vi "bangBangMove.vi"(10 "numRoundingPts":u16, 11 "numPts":u16) -> (3 "roundedHalfTriangle":dbl[](array[numeric]))   [LabVIEW 2016]
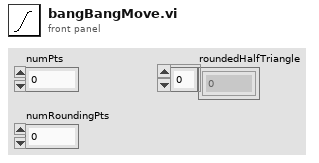
[diagram p1: front panel]
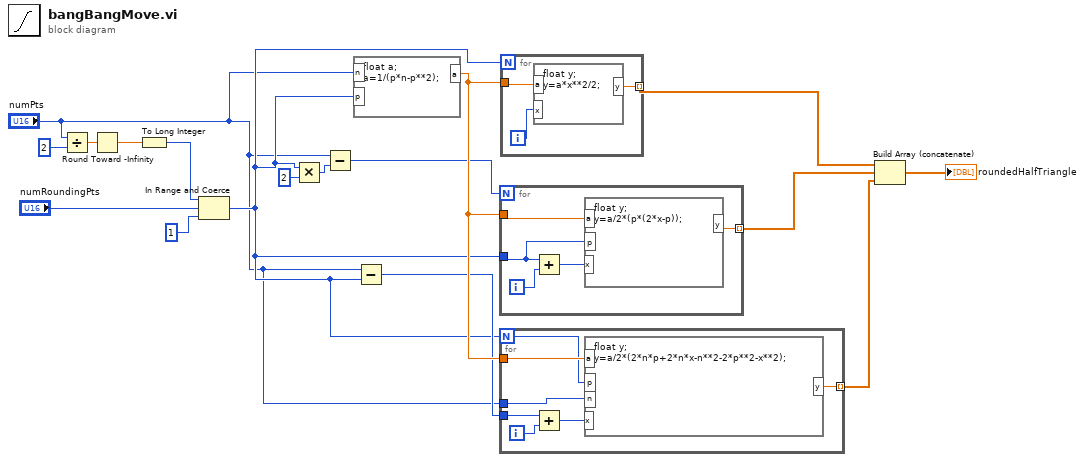
[diagram p0: block diagram]
diagram:
  n1 = Divide(x="numPts", y=u16 2) -> (x/y=w4:dbl)
  n2 = Round Toward -Infinity(1:w4) -> (0:w3:dbl)
  n3 = To Long Integer(number=w3) -> (32bit integer=w1:i32)
  n4 = In Range and Coerce(upper limit=w1, x="numRoundingPts", lower limit=1) -> (coerced(x)=w7:i32)  [unwired: 1 out]
  n5 = Multiply(x=w7, y=u16 2) -> (x*y=w9:i32)
  n6 = Subtract(x="numPts", y=w9) -> (x-y=w10:i32)
  n7 = formula code="float a;\na=1/(p*n-p**2);"("n"="numPts", "p"=w7) -> ("a"=w14:dbl)
  n8 = Subtract(x="numPts", y=w7) -> (x-y=w13:i32)
  n9 = for {
    N: w10 -> [_]
    tunnel: w14 -> [w22]
    tunnel: [w20] -> w12 mode=indexing
    tunnel: w7 -> [w18]
    i -> [w21]
    n10 = Add(x=w18, y=w21) -> (x+y=w19:i32)
    n11 = formula code="float y;\ny=a/2*(p*(2*x-p));"("a"=w22, "x"=w19, "p"=w18) -> ("y"=w20:dbl)
  }
  n12 = for {
    N: w7 -> [w23]
    tunnel: w14 -> [w29]
    tunnel: [w27] -> w15 mode=indexing
    tunnel: w13 -> [w25]
    tunnel: "numPts" -> [w24]
    i -> [w28]
    n13 = Add(x=w25, y=w28) -> (x+y=w26:i32)
    n14 = formula code="float y;\ny=a/2*(2*n*p+2*n*x-n**2-2*p**2-x**2);"("a"=w29, "x"=w26, "n"=w24, "p"=w23) -> ("y"=w27:dbl)
  }
  n15 = for {
    N: w7 -> [_]
    tunnel: w14 -> [w32]
    tunnel: [w30] -> w11 mode=indexing
    i -> [w31]
    n16 = formula code="float y;\ny=a*x**2/2;"("a"=w32, "x"=w31) -> ("y"=w30:dbl)
  }
  n17 = Build Array (concatenate)(w11, w12, w15) -> (→"roundedHalfTriangle":dbl[])
